vi "Ticks to Angel(SubVI).vi"(11 "Numeric in":dbl) -> (3 "Numeric out":dbl)   [LabVIEW 2018, in "Elevator.lvlib" / "Elevator Concrete.lvclass"]
doc: "Use this VI used to convert from 360 degrees to 4096 ticks"
uses:
  Elevator Concrete.lvclass
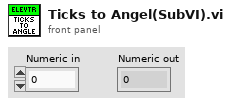
[diagram p1: front panel]
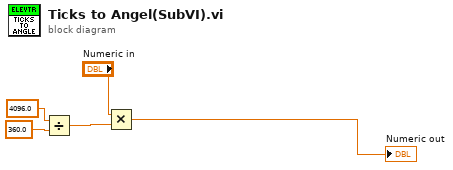
[diagram p0: block diagram]
diagram:
  n1 = Divide(x=4096.0, y=360.0) -> (x/y=w1:dbl)
  n2 = Multiply(x="Numeric in", y=w1) -> (x*y=→"Numeric out":dbl)
